vi "Fetch State Selector.vi"(1 "Close Threshold":dbl, 2 "Perp. Dist.":dbl) -> (0 "State":enum16{"Far", "Close", "Stop"}(ring))   [LabVIEW 2013]
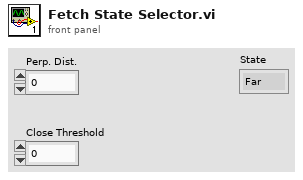
[diagram p1: front panel]
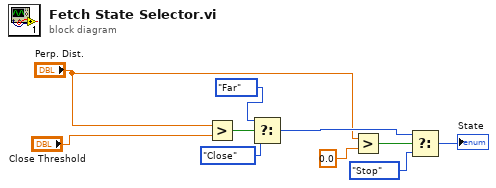
[diagram p0: block diagram]
diagram:
  n1 = Greater?(x="Perp. Dist.", y="Close Threshold") -> (0:w10:bool)
  n2 = Select(t=enum16{"Far", "Close", "Stop"}."Far", s=w10, f=enum16{"Far", "Close", "Stop"}."Close") -> (s? t:f=w6:enum16{"Far", "Close", "Stop"})
  n3 = Greater?(x="Perp. Dist.", y=0.0) -> (0:w7:bool)
  n4 = Select(t=w6, s=w7, f=enum16{"Far", "Close", "Stop"}."Stop") -> (s? t:f=→"State":enum16{"Far", "Close", "Stop"})
